vi "ClusterItemChanged.vi"(10 "NewVal":T1 {"Tons of Peanuts" scale=0.0..10.0}, 11 "OldVal":T1 {"Tons of Peanuts" scale=0.0..10.0}) -> (3 "Numeric":i32)   [LabVIEW 2020]
uses:
  Controls/CLD 16 Control Panel.ctl
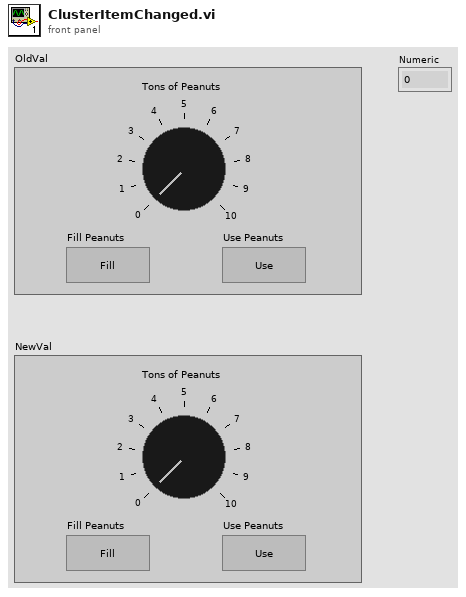
[diagram p1: front panel]
types:
  T1 = typedef "CLD 16 Control Panel.ctl" = cluster{"Tons of Peanuts":i8, "Fill Peanuts":bool, "Use Peanuts":bool}
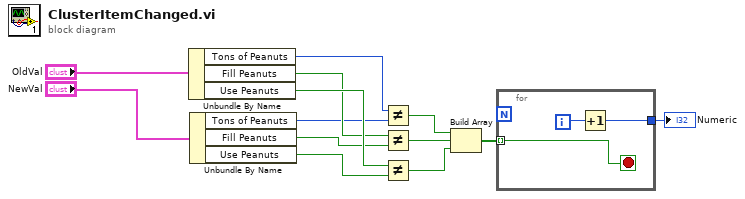
[diagram p0: block diagram]
diagram:
  n1 = Unbundle By Name("OldVal") -> ("Tons of Peanuts"=w3:i8, "Fill Peanuts"=w5:bool, "Use Peanuts"=w7:bool)
  n2 = Unbundle By Name("NewVal") -> ("Tons of Peanuts"=w4:i8, "Fill Peanuts"=w6:bool, "Use Peanuts"=w8:bool)
  n3 = Not Equal?(x=w3, y=w4) -> (x != y?=w9:bool)
  n4 = Not Equal?(x=w5, y=w6) -> (x != y?=w10:bool)
  n5 = Not Equal?(x=w7, y=w8) -> (x != y?=w11:bool)
  n6 = Build Array(w9, w10, w11) -> (w12:bool[])
  n7 = for {
    tunnel: w12 -> [w16] mode=indexing
    tunnel: [w14] -> w13
    i -> [w15]
    stop <- w16 stop-if-true
    n8 = Increment(x=w15) -> (x+1=w14:i32)
  }
  "Numeric" <- w13
